vi "SpkCycle.vi"(7 "LVWSR":refnum<class "Web Request.lvclass">, 9 "auto":u8, 10 "length":u16, 11 "period":u16) -> ()   [LabVIEW 2017]
uses:
  Controller/Messages/Forward Command/Forward Command MSG.lvclass
  <vilib>/MSR Consulting, LLC/General Reuse/PAS/Commands/Change Speaker Cycle Params/Change Speaker Cycle Params.lvclass
  <vilib>/ActorFramework/Message Enqueuer/Message Enqueuer.lvclass
  <vilib>/wsapi/Web Request.lvclass
  Controller/gController.lvclass
  <vilib>/MSR Consulting, LLC/General Reuse/Command/Command.lvclass
  C:/Program Files (x86)/National Instruments/LabVIEW 2017/vi.lib/ActorFramework/Message/Message.lvclass
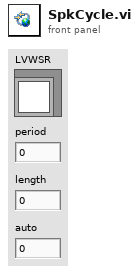
[diagram p1: front panel]
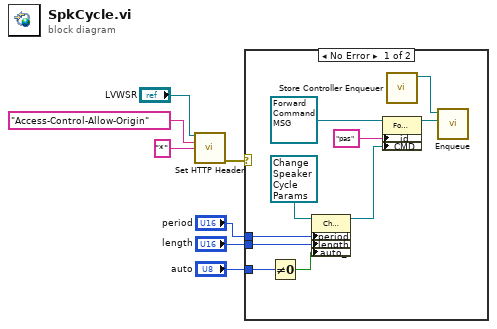
[diagram p0: block diagram]
diagram:
  n1 = call <vilib>:"Set HTTP Header.vi"("LabVIEW Web Service Request"="LVWSR", "header"="Access-Control-Allow-Origin", "header value"="*") -> ("error out"=w1:errorcluster)  [unwired: 11 in, 1 out]
  n2 = case shown="No Error" w1 {
    tunnel: "period" -> [w13 _]
    tunnel: "length" -> [w12 _]
    tunnel: "auto" -> [w11 _]
    frame No Error {
      n3 = Not Equal To 0?(x=w11) -> (x != 0?=w10:bool)
      n4 = property class="Change Speaker Cycle Params.lvc"(reference=refnum<class "Change Speaker Cycle Params.lvclass"> refnum ("PAS Library.lvlib:Change Speaker Cycle Params"), "period"=w13, "length"=w12, "auto_"=w10) -> (reference out=w14:refnum<class "Change Speaker Cycle Params.lvclass">)  [unwired: 1 in, 1 out]
      n5 = property class="Forward Command MSG"(reference=refnum<class "Forward Command MSG.lvclass"> refnum ("Controller.lvlib:Forward Command MSG"), "id"="pas", "CMD"=w14) -> (reference out=w9:refnum<class "Forward Command MSG.lvclass">)  [unwired: 1 in, 1 out]
      n6 = call "Store Controller Enqueuer.vi"() -> ("Controller Enqueuer Out"=w8:refnum<class "Message Enqueuer.lvclass">)  [unwired: 11 in]
      n7 = call <vilib>:"Enqueue.vi"("Message"=w9, "Message Enqueuer in"=w8) -> ()  [unwired: 8 in, 2 out]
    }
    frame Error {
    }
  }
